vi "Get Class Image Index.vi"(8 "error in (no error)":errorcluster, 10 "SerializableObject in":refnum<class "SerializableObject.lvclass">, 11 "Editor.lvclass in":refnum<data-value>) -> (0 "error out":errorcluster, 1 "Index":i32, 2 "SerializableObject out":refnum<class "SerializableObject.lvclass">, 3 "Editor.lvclass out":refnum<data-value>)   [LabVIEW 2015, in "Editor.lvclass"]
uses:
  Editor.lvclass
  SerializableObject/SerializableObject.lvclass
  <vilib>/picture/picture.llb/imagedata.ctl
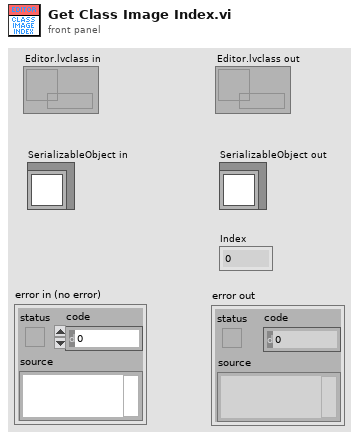
[diagram p1: front panel]
types:
  T1 = typedef "imagedata.ctl" = cluster{"image type":i32, "image depth":i32, "image":u8[], "mask":u8[], "colors":u32[], "Rectangle":cluster{"left":i16, "top":i16, "right":i16, "bottom":i16}}
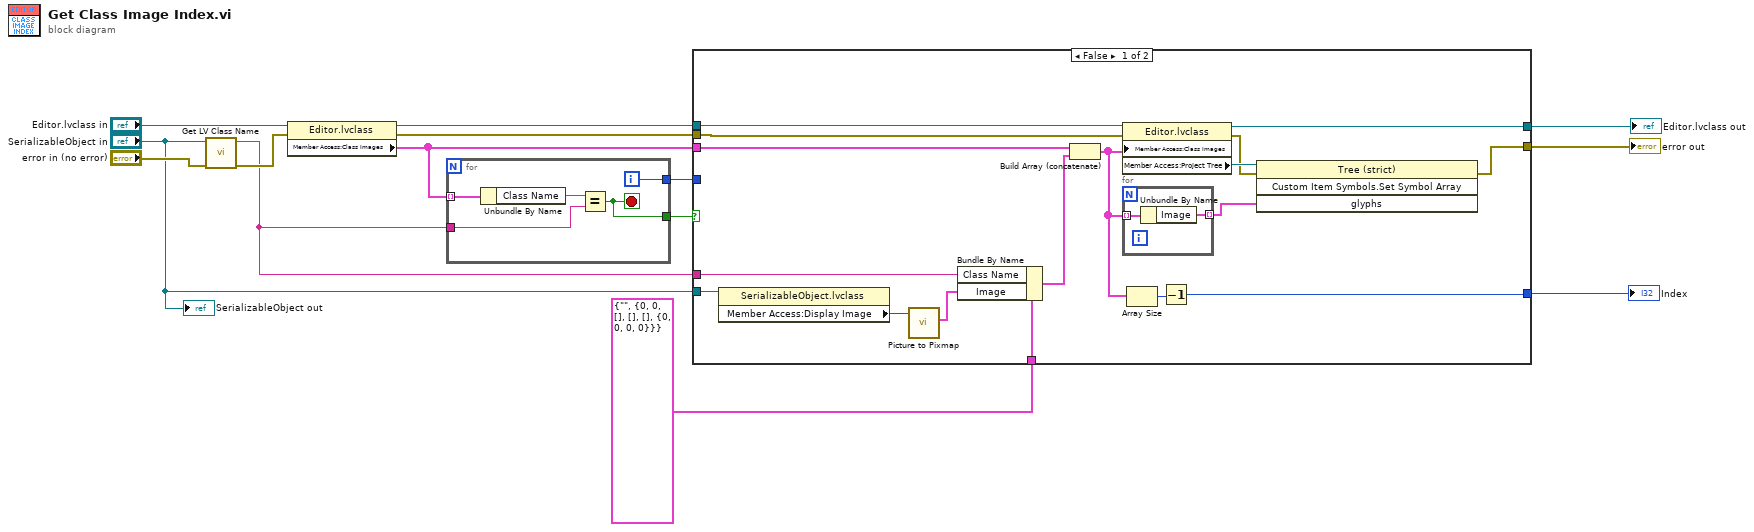
[diagram p0: block diagram]
diagram:
  n1 = call <vilib>:"Get LV Class Name.vi"("error in (no error)"="error in (no error)", "object"="SerializableObject in") -> ("error out"=w7:errorcluster, "class name"=w6:string)  [unwired: 8 in]
  n2 = property class="Editor.lvclass"(reference="Editor.lvclass in", error in=w7) -> (reference out=w9:refnum<data-value>, error out=w10:errorcluster, "Member Access:Class Images"=w5:cluster{"Class Name":string, "Image":T1}[])
  n3 = for {
    tunnel: w5 -> [w19] mode=indexing
    tunnel: w6 -> [w17]
    tunnel: [w16] -> w13
    tunnel: [w15] -> w12
    i -> [w15]
    stop <- w16 stop-if-true
    n4 = Unbundle By Name(w19) -> ("Class Name"=w18:string)
    n5 = Equal?(x=w18, y=w17) -> (x = y?=w16:bool)
  }
  n6 = case shown="False" w13 {
    tunnel: w12 -> [_ w41]
    tunnel: [w27 w41] -> w11
    tunnel: w10 -> [w30 w39]
    tunnel: w9 -> [w31 w40]
    tunnel: "SerializableObject in" -> [w36 _]
    tunnel: w6 -> [w34 _]
    tunnel: w5 -> [w33 _]
    tunnel: cluster{"Class Name":string, "Image":T1} {"Class Name"="", "Image"={"image type"=0, "image depth"=0, "image"=[], "mask"=[], "colors"=[], "Rectangle"={"left"=0, "top"=0, "right"=0, "bottom"=0}}} -> [w35 _]
    tunnel: [w29 w40] -> w3
    tunnel: [w22 w39] -> w2
    frame False {
      n7 = property class="SerializableObject.lvclass"(reference=w36) -> ("Member Access:Display Image"=w20:picture)  [unwired: 1 in, 2 out]
      n8 = call <vilib>:"Picture to Pixmap.vi"("picture"=w20) -> ("image data"=w21:T1)  [unwired: 9 in, 1 out]
      n9 = Bundle By Name(cluster=w35, "Class Name"=w34, "Image"=w21) -> (w32:cluster{"Class Name":string, "Image":T1})
      n10 = Build Array (concatenate)(w33, w32) -> (w26:cluster{"Class Name":string, "Image":T1}[])
      n11 = property class="Editor.lvclass"(reference=w31, error in=w30, "Member Access:Class Images"=w26) -> (reference out=w29:refnum<data-value>, error out=w23:errorcluster, "Member Access:Project Tree"=w25:refnum<vi>)
      n12 = for {
        tunnel: w26 -> [w38] mode=indexing
        tunnel: [w37] -> w24 mode=indexing
        n13 = Unbundle By Name(w38) -> ("Image"=w37:T1)
      }
      n14 = Array Size(array=w26) -> (size(s)=w28:i32)
      n15 = Decrement(x=w28) -> (x-1=w27:i32)
      n16 = invoke class="Tree (strict)" method="Custom Item Symbols.Set Symbol Array"(reference=w25, error in=w23, "glyphs"=w24) -> (error out=w22:errorcluster)  [unwired: 1 in, 3 out]
    }
    frame True {
    }
  }
  "error out" <- w2
  "Index" <- w11
  "Editor.lvclass out" <- w3
  "SerializableObject out" <- "SerializableObject in"
